vi "cv.to.local_issue.vi"(8 "error in (no error)":errorcluster, 11 "cv_issue":T5) -> (0 "error out":errorcluster, 3 "local_issue":T1 {"display_date" format="%<%x>T"})   [LabVIEW 2024, in "CV_RESTful_Lib.lvlib"]
uses:
  CV_RESTful_Lib.lvlib
  typedefs/cv_issue--cluster.ctl
  typedefs/cv_issue.results--cluster.ctl
  typedefs/cv_issue.associated_image--cluster.ctl
  typedefs/cv_issue.generic_credit--cluster.ctl
  typedefs/cv_issue.person_credit--cluster.ctl
  typedefs/local_issue--cluster.ctl
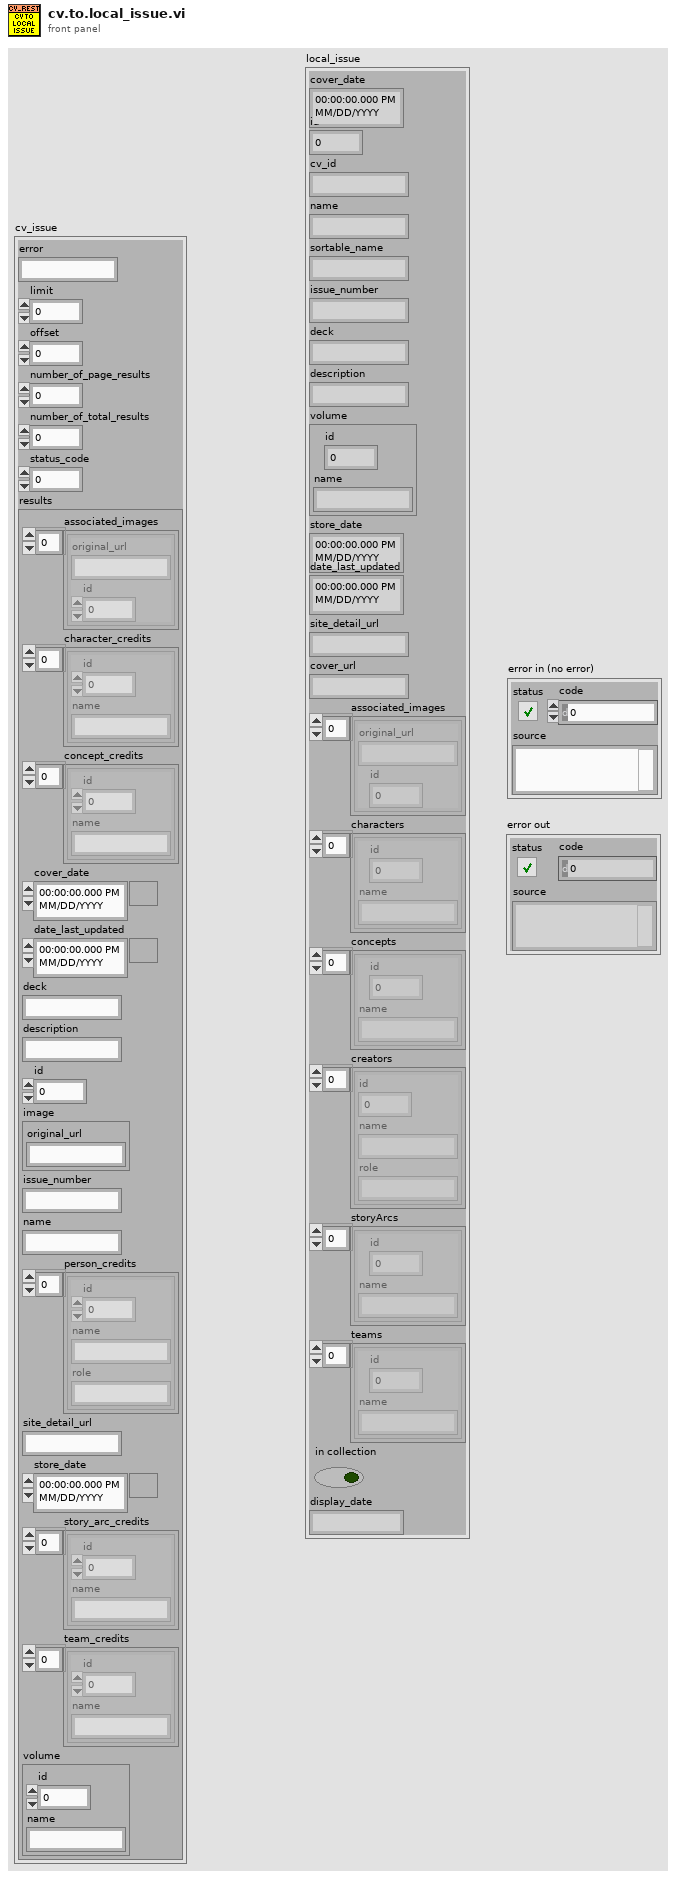
[diagram p1: front panel]
types:
  T1 = typedef "CV_RESTful_Lib.lvlib/local_issue--cluster.ctl" = cluster{"cover_date":timestamp, "id":i32, "cv_id":string, "name":string, "sortable_name":string, "issue_number":string, "deck":string, "description":string, "volume":T2, "store_date":timestamp, "date_last_updated":timestamp, "site_detail_url":string, "cover_url":string, "associated_images":T3[], "characters":T2[], "concepts":T2[], "creators":T4[], "storyArcs":T2[], "teams":T2[], "in collection":bool, "display_date":timestamp}
  T2 = typedef "CV_RESTful_Lib.lvlib/cv_issue.generic_credit--cluster.ctl" = cluster{"id":i32, "name":string}
  T3 = typedef "CV_RESTful_Lib.lvlib/cv_issue.associated_image--cluster.ctl" = cluster{"original_url":string, "id":i32}
  T4 = typedef "CV_RESTful_Lib.lvlib/cv_issue.person_credit--cluster.ctl" = cluster{"id":i32, "name":string, "role":string}
  T5 = typedef "CV_RESTful_Lib.lvlib/cv_issue--cluster.ctl" = cluster{"error":string, "limit":i32, "offset":i32, "number_of_page_results":i32, "number_of_total_results":i32, "status_code":i32, "results":T6}
  T6 = typedef "CV_RESTful_Lib.lvlib/cv_issue.results--cluster.ctl" = cluster{"associated_images":T3[], "character_credits":T2[], "concept_credits":T2[], "cover_date":timestamp, "date_last_updated":timestamp, "deck":string, "description":string, "id":i32, "image":cluster{"original_url":string}, "issue_number":string, "name":string, "person_credits":T4[], "site_detail_url":string, "store_date":timestamp, "story_arc_credits":T2[], "team_credits":T2[], "volume":T2}
  T7 = typedef "LVDateTimeRec.ctl" = cluster{"fractional second":dbl, "second":i32, "minute":i32, "hour":i32, "day of month":i32, "month":i32, "year":i32, "day of week":i32, "day of year":i32, "DST":i32}
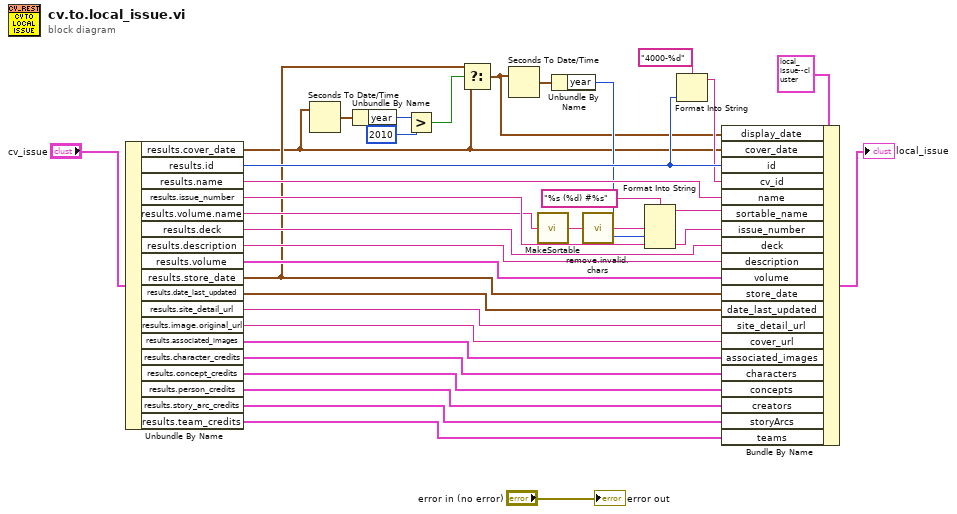
[diagram p0: block diagram]
diagram:
  n1 = Unbundle By Name("cv_issue") -> ("results.cover_date"=w1:timestamp, "results.id"=w31:i32, "results.name"=w26:string, "results.issue_number"=w22:string, "results.volume.name"=w8:string, "results.deck"=w21:string, "results.description"=w20:string, "results.volume"=w19:T2, "results.store_date"=w3:timestamp, "results.date_last_updated"=w18:timestamp, "results.site_detail_url"=w17:string, "results.image.original_url"=w16:string, "results.associated_images"=w15:T3[], "results.character_credits"=w14:T2[], "results.concept_credits"=w13:T2[], "results.person_credits"=w12:T4[], "results.story_arc_credits"=w11:T2[], "results.team_credits"=w10:T2[])
  n2 = Seconds To Date/Time(time stamp (now)=w1) -> (date time rec=w7:T7)  [unwired: 1 in]
  n3 = Unbundle By Name(w7) -> ("year"=w6:i32)
  n4 = Greater?(x=w6, y=2010) -> (0:w4:bool)
  n5 = Select(t=w3, s=w4, f=w1) -> (s? t:f=w2:timestamp)
  n6 = Seconds To Date/Time(time stamp (now)=w2) -> (date time rec=w24:T7)  [unwired: 1 in]
  n7 = call "MakeSortable.vi"("string in"=w8) -> ("string out"=w29:string)
  n8 = Unbundle By Name(w24) -> ("year"=w23:i32)
  n9 = call "remove.invalid.chars.vi"("string in"=w29) -> ("string out"=w27:string)
  n10 = Format Into String(format string="%s (%d) #%s", w27, w23, w22) -> (resulting string=w25:string)  [unwired: 2 in, 1 out]
  n11 = Format Into String(format string="4000-%d", w31) -> (resulting string=w30:string)  [unwired: 2 in, 1 out]
  n12 = Bundle By Name(cluster=T1 {"cover_date"=timestamp(0 s since 1904-01-01), "id"=0, "cv_id"="", "name"="", "sortable_name"="", "issue_number"="", "deck"="", "description"="", "volume"={"id"=0, "name"=""}, "store_date"=timestamp(0 s since 1904-01-01), "date_last_updated"=timestamp(0 s since 1904-01-01), "site_detail_url"="", "cover_url"="", "associated_images"=[], "characters"=[], "concepts"=[], "creators"=[], "storyArcs"=[], "teams"=[], "in collection"=FALSE, "display_date"=timestamp(0 s since 1904-01-01)} ("local_issue"), "display_date"=w2, "cover_date"=w1, "id"=w31, "cv_id"=w30, "name"=w26, "sortable_name"=w25, "issue_number"=w22, "deck"=w21, "description"=w20, "volume"=w19, "store_date"=w3, "date_last_updated"=w18, "site_detail_url"=w17, "cover_url"=w16, "associated_images"=w15, "characters"=w14, "concepts"=w13, "creators"=w12, "storyArcs"=w11, "teams"=w10) -> (→"local_issue":T1)
  "error out" <- "error in (no error)"
